vi "PL_Global.vi"() -> ()   [LabVIEW 2020]
panel:
  in  "Cluster":T1
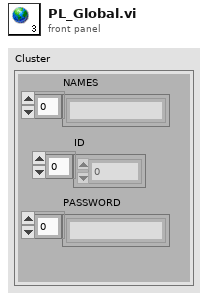
[diagram p1: front panel]
types:
  T1 = cluster{"NAMES":string[], "ID":dbl[], "PASSWORD":string[]}
diagram:
